vi "Load File.vi"() -> ()   [LabVIEW 2025]
uses:
  <vilib>/Utility/file.llb/Read Delimited Spreadsheet (DBL).vi
panel:
  out "After Outlier Removal":dbl[](graph)
  in  "Z Threshold":dbl
  in  "Data File Path":path
  out "Time vs Signal":waveform(dbl)(graph)
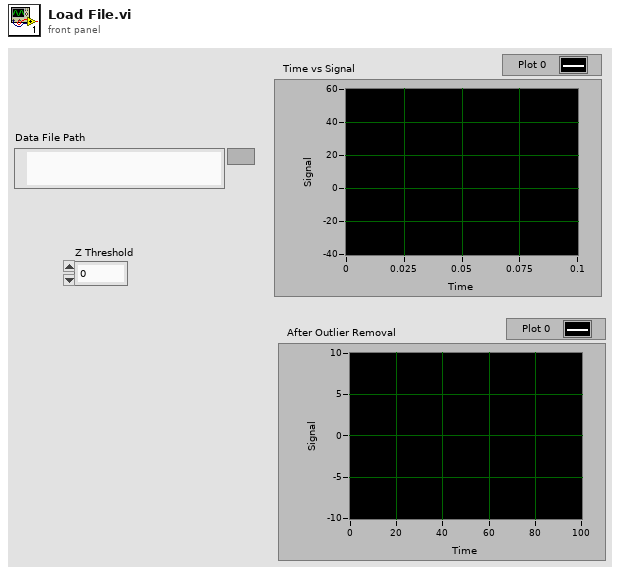
[diagram p1: front panel]
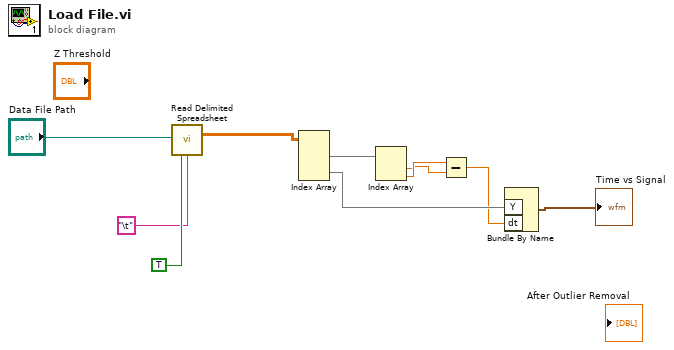
[diagram p0: block diagram]
diagram:
  n1 = call-poly <vilib>:"Read Delimited Spreadsheet.vi"("file path (dialog if empty)"="Data File Path", "transpose? (F)"=TRUE, "delimiter (\\t)"="\t" ("delimiter (\\t)")) -> ("all rows"=w8:dbl[][])  [unwired: 7 in, 5 out]
  n2 = Index Array(array=w8) -> (element #1=w7:dbl[], element #2=w3:dbl[])  [unwired: 4 in]
  n3 = Index Array(array=w7) -> (element #1=w5:dbl, element #2=w6:dbl)  [unwired: 2 in]
  n4 = Subtract(x=w6, y=w5) -> (x-y=w2:dbl)
  n5 = Bundle By Name("Y"=w3, "dt"=w2) -> (→"Time vs Signal":waveform(dbl))  [unwired: 1 in]
